vi "Stop Generation.vi"(8 "error in (no error)":errorcluster, 11 "Hardware Resources in":T1={"AO"={"task name"="AO", "task_ref"="", "physical channels"="Dev1/ao0"}, "PID"={"P"=0.0, "I"=0.0, "D"=0.0}, "conversions"={"ao0"={"a"=0.0, "b"=0.0}}, "setpoint"=0.0}) -> (0 "error out":errorcluster)   [LabVIEW 2014, in "PLS Generation.lvlib"]
doc: "Stops the acquisition."
uses:
  PLS Generation.lvlib
  Hardware Configuration.ctl
  Settings/conversion.ctl
  Settings/PLS Settings.lvlib
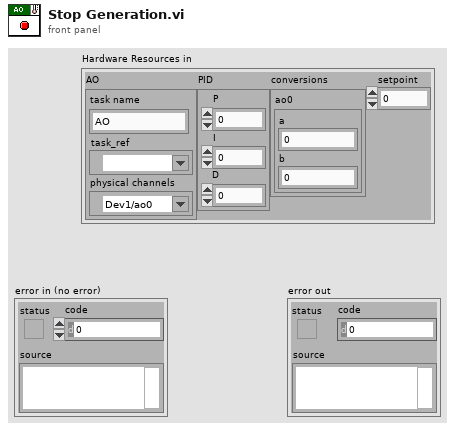
[diagram p1: front panel]
types:
  T1 = typedef "PLS Generation.lvlib/Hardware Configuration.ctl" = cluster{"AO":cluster{"task name":string, "task_ref":refnum<k21>, "physical channels":tag}, "PID":cluster{"P":dbl, "I":dbl, "D":dbl}, "conversions":cluster{"ao0":T2}, "setpoint":dbl}
  T2 = typedef "PLS Settings.lvlib/conversion.ctl" = cluster{"a":dbl, "b":dbl}
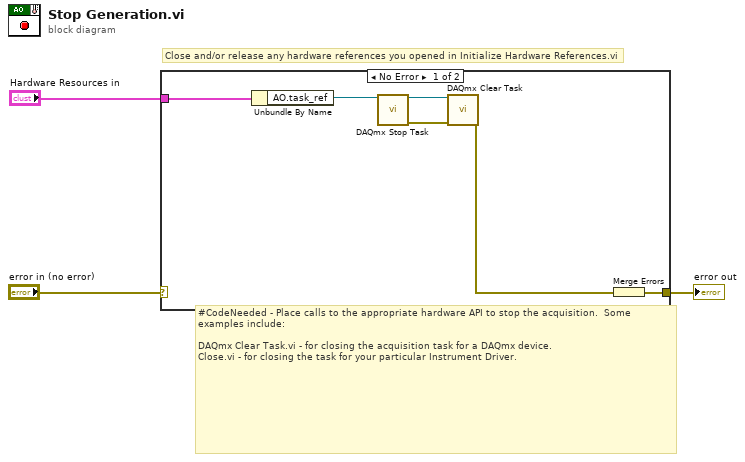
[diagram p0: block diagram]
diagram:
  # "#CodeNeeded - Place calls to the appropriate hardware API to stop the acquisition.  Some examples include:\n\nDAQmx Clear Task.vi - for closing the acquisition task for a DAQmx device.\nClose.vi - for closing the task for your particular Instrument Driver."
  # "Close and/or release any hardware references you opened in Initialize Hardware References.vi"
  n1 = case shown="No Error" "error in (no error)" {
    selector: "error in (no error)" -> [_ w10]
    tunnel: [w9 w10] -> w2
    tunnel: "Hardware Resources in" -> [w8 _]
    frame No Error {
      n2 = Unbundle By Name(w8) -> ("AO.task_ref"=w7:refnum<k21>)
      n3 = call <vilib>:"DAQmx Stop Task.vi"("task/channels in"=w7) -> ("task out"=w6:refnum<k21>, "error out"=w5:errorcluster)  [unwired: 13 in]
      n4 = call <vilib>:"DAQmx Clear Task.vi"("task in"=w6, "error in"=w5) -> ("error out"=w4:errorcluster)  [unwired: 13 in]
      n5 = Merge Errors(w4) -> (w9:errorcluster)
    }
    frame Error {
    }
  }
  "error out" <- w2
